vi "GetUIRef.vi"(0 "reference in":refnum<class "GUI.lvclass">, 11 "error in (no error)":errorcluster) -> (4 "reference out":refnum<class "GUI.lvclass">, 6 "UI VI":refnum<vi>, 15 "error out":errorcluster)   [LabVIEW 2019]
uses:
  GUI.lvclass
  D:/LabASF/LabASF/src/Proccess_class/Proccess.lvclass
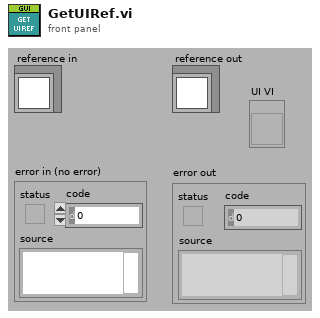
[diagram p1: front panel]
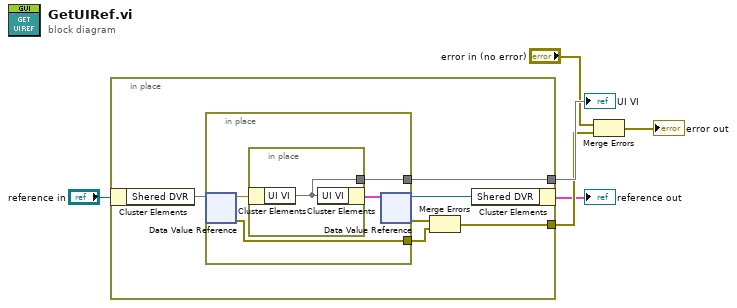
[diagram p0: block diagram]
diagram:
  n1 = in-place {
    in-place-border: [w8] -> w4
    in-place-border: [w7] -> w5
    n2 = in-place-cluster #1("reference in") -> ("Shered DVR"=w12)
    n3 = in-place {
      in-place-border: [w14] -> w9
      in-place-border: [w13] -> w7
      n4 = in-place-dvr #2(w12) -> (w16:dbl, w14:errorcluster)
      n5 = in-place {
        in-place-border: [w17] -> w13
        n6 = in-place-cluster #3(w16) -> ("UI VI"=w17)
        n7 = in-place-cluster #3("UI VI"=w17) -> (w15:cluster{})
      }
      n8 = in-place-dvr #2(w15) -> (w11:refnum<data-value>, w10:errorcluster)
    }
    n9 = Merge Errors(w10, w9) -> (w8:errorcluster)
    n10 = in-place-cluster #1("Shered DVR"=w11) -> (→"reference out":cluster{})
  }
  "UI VI" <- w5
  n11 = Merge Errors("error in (no error)", w4) -> (→"error out":errorcluster)
